vi "Swerve.vi"(7 "Description":string, 8 "Command Info In":T3, 11 "SubSystem Data":T1) -> (0 "Command Info Out":T3)   [LabVIEW 2020]
doc: "This template is useful for immediate subsystem actions that do not need deadband filtering\n\nBe sure to right-click and select New from Template and save with a new command name."
uses:
  <vilib>/Rock Robotics/WPI/Framework/Command Status Info.ctl
  <vilib>/Rock Robotics/WPI/Framework/Completion Status.ctl
  <vilib>/Rock Robotics/WPI/Framework/Completion Notifier.ctl
  Implementation/Swerve Setpoints.ctl
  Implementation/Swerve Operations.ctl
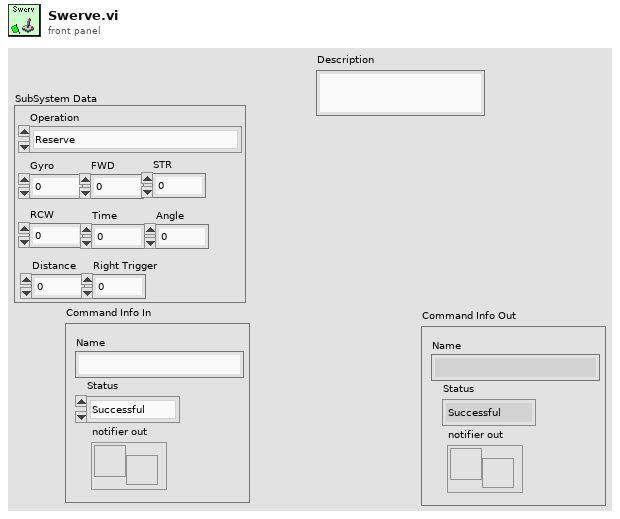
[diagram p1: front panel]
types:
  T1 = typedef "Swerve Setpoints.ctl" = cluster{"Operation":T2, "Gyro":dbl, "RCW":dbl, "FWD":dbl, "STR":dbl, "Time":dbl, "Angle":dbl, "Distance":dbl, "Right Trigger":dbl}
  T2 = typedef "Swerve Operations.ctl" = enum16{"Reserve", "Read Current", "Immediate", "Joystick Drive", "Drive for Distance", "Drive for Time", "Turn to Angle", "Drive to Angle(Time)", "Drive to Angle(Distance)"}
  T3 = typedef "Command Status Info.ctl" = cluster{"Name":string, "Status":T4, "notifier out":T5}
  T4 = typedef "Completion Status.ctl" = enum16{"Successful", "Aborted", "Incomplete"}
  T5 = typedef "Completion Notifier.ctl" = refnum<notifier>
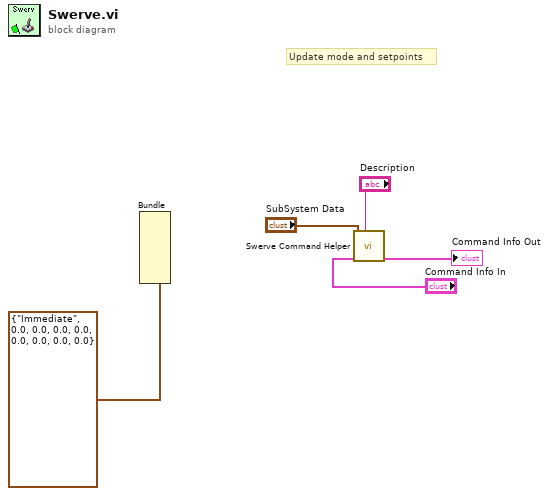
[diagram p0: block diagram]
diagram:
  # "Update mode and setpoints"
  n1 = Bundle(cluster=T1 {"Operation"=enum."Immediate", "Gyro"=0.0, "RCW"=0.0, "FWD"=0.0, "STR"=0.0, "Time"=0.0, "Angle"=0.0, "Distance"=0.0, "Right Trigger"=0.0} ("SubSystem Data")) -> ()  [unwired: 9 in, 1 out]
  n2 = call "Swerve Command Helper.vi"("Description"="Description", "Command Info In"="Command Info In", "SubSystem Data"="SubSystem Data") -> ("Command Info Out"=→"Command Info Out":T3)  [unwired: 6 in, 2 out]
